vi "Unsubscribe.vi"(8 "error in (no error)":errorcluster, 10 "Key":string="myhome/kitchen/temp", 11 "Zenoh in":refnum<class "Zenoh.lvclass">) -> (0 "error out":errorcluster, 3 "Zenoh out":refnum<class "Zenoh.lvclass">)   [LabVIEW 2021, in "Zenoh.lvclass"]
uses:
  Zenoh.lvclass
  Zenoh.lvclass/Zenoh.ctl
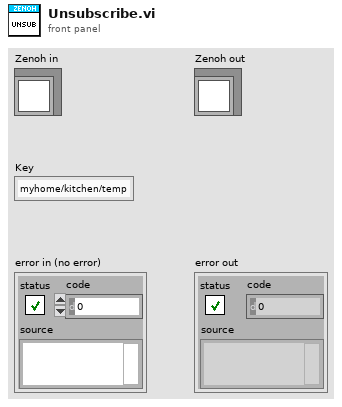
[diagram p1: front panel]
types:
  T1 = typedef "Zenoh.lvclass/Channel Info.ctl" = cluster{"Mime Type":string, "Reader Handle":i64}
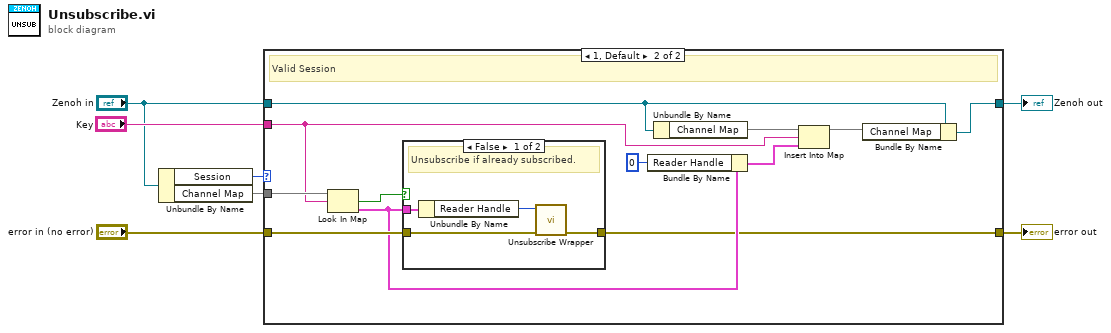
[diagram p0: block diagram]
diagram:
  n1 = Unbundle By Name("Zenoh in") -> ("Session"=w3:i64, "Channel Map"=w4:map{string, T1})
  n2 = case shown="1, Default" w3 {
    tunnel: "Key" -> [_ w10]
    tunnel: "error in (no error)" -> [w8 w21]
    tunnel: "Zenoh in" -> [w9 w18]
    tunnel: w4 -> [_ w20]
    tunnel: [w8 w16] -> w2
    tunnel: [w9 w15] -> w1
    frame 0 {
      # "Invalid session"
    }
    frame 1, Default {
      # "Valid Session"
      n3 = Look In Map(map=w20, key=w10) -> (key not found?=w19:bool, value=w17:T1)  [unwired: 1 in]
      n4 = case shown="False" w19 {
        tunnel: w21 -> [w25 w26]
        tunnel: w17 -> [w24 _]
        tunnel: [w22 w26] -> w16
        frame False {
          # "Unsubscribe if already subscribed."
          n5 = Unbundle By Name(w24) -> ("Reader Handle"=w23:i64)
          n6 = call "Unsubscribe Wrapper.vi"("error in (no error)"=w25, "Reader Handle"=w23) -> ("error out"=w22:errorcluster)  [unwired: 9 in]
        }
        frame True {
        }
      }
      n7 = Bundle By Name(cluster=w17, "Reader Handle"=i64 0) -> (w13:T1)
      n8 = Unbundle By Name(w18) -> ("Channel Map"=w14:map{string, T1})
      n9 = Insert Into Map(map in=w14, key=w10, value=w13) -> (map out=w12:map{string, T1})  [unwired: 2 out]
      n10 = Bundle By Name(cluster=w18, "Channel Map"=w12) -> (w15:refnum<class "Zenoh.lvclass">)
    }
  }
  "error out" <- w2
  "Zenoh out" <- w1
